vi "simmer.vi"(8 "error in (no error)":errorcluster, 11 "HotPlate in":refnum<class "HotPlate.lvclass">) -> (0 "error out":errorcluster, 3 "HotPlate out":refnum<class "HotPlate.lvclass">)   [LabVIEW 2011, in "HotPlate.lvclass"]
uses:
  HotPlate.lvclass
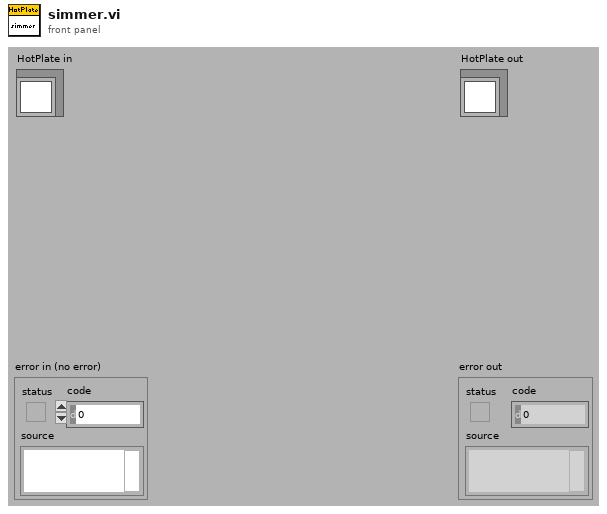
[diagram p1: front panel]
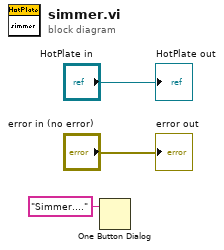
[diagram p0: block diagram]
diagram:
  n1 = One Button Dialog(message="Simmer....") -> ()  [unwired: 1 in, 1 out]
  "error out" <- "error in (no error)"
  "HotPlate out" <- "HotPlate in"
